vi "ClientPool_CreateDestroyAndRecreateClients_ClientsCreatedWithDifferentGrpcId.vi"(8 "error in (no error)":errorcluster) -> (0 "error out":errorcluster, 2 "result":string, 3 "pass":bool)   [LabVIEW 2020, in "MeasurementServerTests.lvlib"]
uses:
  MeasurementServerTests.lvlib
  Runtime/MeasurementLink Measurement Server/Classes/GrpcClientPool/FGV Action.ctl
  Runtime/MeasurementLink Measurement Server/Classes/GrpcClientPool/GrpcClientPool.lvclass
panel:
  in  "Action":T1
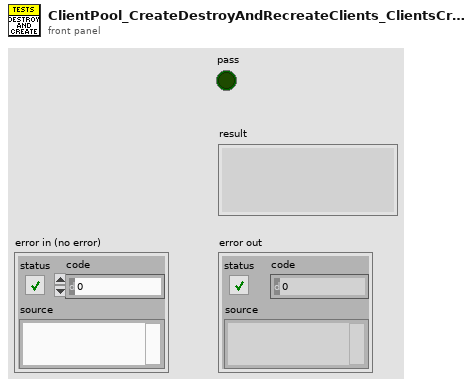
[diagram p1: front panel]
types:
  T1 = typedef "MeasurementLink Measurement Server.lvlib/GrpcClientPool.lvclass/FGV Action.ctl" = enum16{"Get Discovery Client", "Get Session Client", "Get Pinmap Client", "Destroy Clients"}
  T2 = typedef "grpc-lvsupport-release.lvlib/grpcId.ctl" = u64
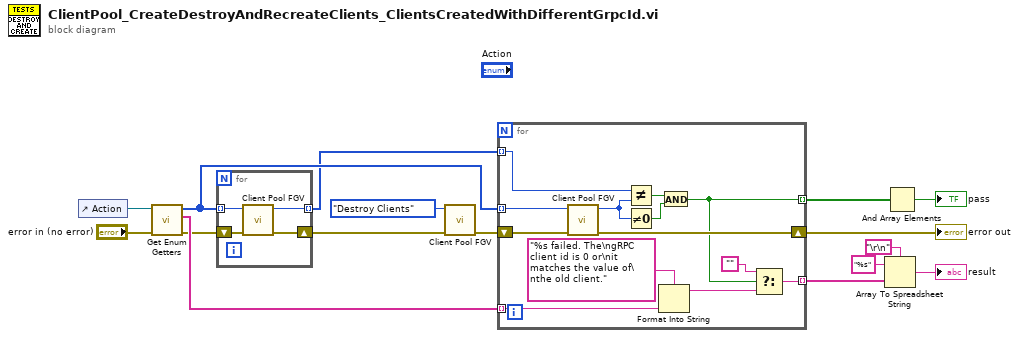
[diagram p0: block diagram]
diagram:
  n1 = control-ref of="Action"() -> (w7:refnum<vi>)
  n2 = call "Get Enum Getters.vi"("error in (no error)"="error in (no error)", "enum ref in"=w7) -> ("error out"=w6:errorcluster, "enum strings"=w12:string[], "enum numbers"=w2:i32[])  [unwired: 7 in]
  n3 = for {
    tunnel: w2 -> [w20] mode=indexing
    shift-right: [w18] -> w5
    shift-left: w6 -> [w19]
    tunnel: [w17] -> w1 mode=indexing
    n4 = call "Client Pool FGV.vi"("error in (no error)"=w19, "Action"=w20) -> ("error out"=w18:errorcluster, "grpc client id"=w17:T2)  [unwired: 8 in]
  }
  n5 = call "Client Pool FGV.vi"("error in (no error)"=w5, "Action"=FGV_Action."Destroy Clients") -> ("error out"=w4:errorcluster)  [unwired: 8 in, 1 out]
  n6 = for {
    shift-right: [w32] -> w16
    shift-left: w4 -> [w33]
    tunnel: w2 -> [w31] mode=indexing
    tunnel: [w21] -> w14 mode=indexing
    tunnel: w12 -> [w30] mode=indexing
    tunnel: [w26] -> w11 mode=indexing
    tunnel: w1 -> [w25] mode=indexing
    n7 = call "Client Pool FGV.vi"("error in (no error)"=w33, "Action"=w31) -> ("error out"=w32:errorcluster, "grpc client id"=w23:T2)  [unwired: 8 in]
    n8 = Not Equal?(x=w25, y=w23) -> (x != y?=w24:bool)
    n9 = Not Equal To 0?(x=w23) -> (x != 0?=w22:bool)
    n10 = Format Into String(format string="%s failed. The\ngRPC client id is 0 or\nit matches the value of\nthe old client." ("result"), w30) -> (resulting string=w28:string)  [unwired: 2 in, 1 out]
    n11 = And(x=w24, y=w22) -> (x .and. y?=w21:bool)
    n12 = Select(t="", s=w21, f=w28) -> (s? t:f=w26:string)
  }
  "error out" <- w16
  n13 = Array To Spreadsheet String(delimiter (Tab)="\r\n", array=w11, 3:"%s" ("format string")) -> (spreadsheet string=→"result":string)
  n14 = And Array Elements(Boolean array=w14) -> (logical AND=→"pass":bool)
